vi "Test Noise Mode.vi"(8 "error in (no error)":errorcluster, 11 "VISA resource name":refnum<visa-resource-name>) -> (0 "error out":errorcluster, 3 "VISA resource name":refnum<visa-resource-name>)   [LabVIEW 2019, in "SR7270 Drivers.lvlib"]
uses:
  SR7270 Drivers.lvlib
  Typedefs/NOISEMODE--enum.ctl
  <vilib>/addons/_JKI Toolkits/Caraya/classes/Assert/Assert.lvclass
  <vilib>/addons/_JKI Toolkits/Caraya/classes/Test/Test.lvclass
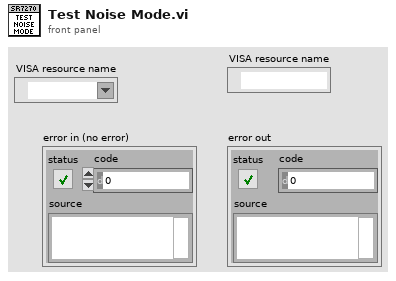
[diagram p1: front panel]
types:
  T1 = typedef "SR7270 Drivers.lvlib/NOISEMODE--enum.ctl" = enum16{"OFF", "ON"}
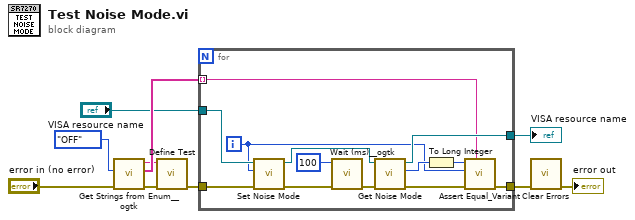
[diagram p0: block diagram]
diagram:
  n1 = call <userlib>:"Get Strings from Enum__ogtk.vi"("error in (no error)"="error in (no error)", "Enum"=NOISEMODE--enum."OFF" ("Noise Measurement Mode")) -> ("error out"=w5:errorcluster, "Enum Strings"=w8:string[], "Enum Name"=w6:string)  [unwired: 6 in, 1 out]
  n2 = call <vilib>:"Define Test.vi"("error in (no error)"=w5, "Label (VI Title)"=w6) -> ("error out"=w3:errorcluster)  [unwired: 9 in]
  n3 = for {
    tunnel: "VISA resource name" -> [w22]
    tunnel: w3 -> [w14]
    tunnel: [w20] -> w10
    tunnel: [w19] -> w1
    tunnel: w8 -> [w11] mode=indexing
    i -> [w13]
    n4 = call "Set Noise Mode.vi"("error in (no error)"=w14, "Noise Measurement Mode"=w13, "VISA resource name"=w22) -> ("error out"=w16:errorcluster, "VISA resource name out"=w23:refnum<visa-resource-name>)  [unwired: 7 in]
    n5 = call <userlib>:"Wait (ms)__ogtk.vi"("error in (no error)"=w16, "milliseconds to wait"=u32 100) -> ("error out"=w18:errorcluster)  [unwired: 8 in, 1 out]
    n6 = call "Get Noise Mode.vi"("error in (no error)"=w18, "VISA resource name"=w23) -> ("error out"=w21:errorcluster, "Noise Measurement Mode"=w15:T1, "VISA resource name out"=w19:refnum<visa-resource-name>)  [unwired: 7 in]
    n7 = To Long Integer(number=w15) -> (32bit integer=w12:i32)
    n8 = call <vilib>:"Assert Equal_Variant.vi"("Label"=w11, "error in (no error)"=w21, "Y"=w13, "X"=w12) -> ("error out"=w20:errorcluster)  [unwired: 7 in]
  }
  "VISA resource name" <- w1
  n9 = call <vilib>:"Clear Errors.vi"("error in (no error)"=w10) -> ("error out"=→"error out":errorcluster)  [unwired: 5 in, 1 out]
